vi "LongTimeToShift.vi"(2 "input string":string) -> (0 "s? t:f":string)   [LabVIEW 2012]
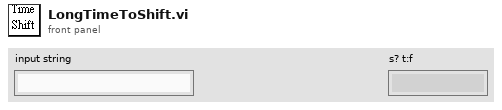
[diagram p1: front panel]
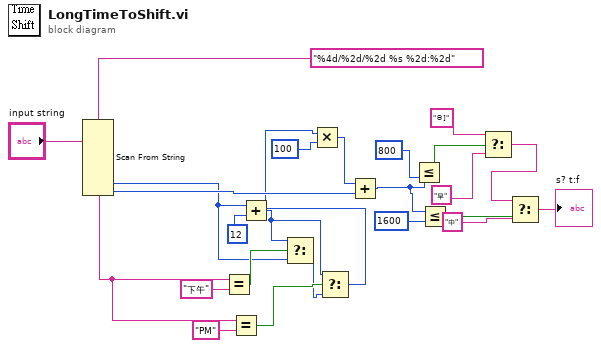
[diagram p0: block diagram]
diagram:
  n1 = Scan From String(format string="%4d/%2d/%2d %s %2d:%2d", input string="input string") -> (output 4=w5:string, output 5=w7:i32, output 6=w11:i32)  [unwired: 11 in, 3 out]
  n2 = Equal?(x=w5, y="下午") -> (x = y?=w9:bool)
  n3 = Equal?(x=w5, y="PM") -> (x = y?=w4:bool)
  n4 = Add(x=w7, y=12) -> (x+y=w2:i32)
  n5 = Select(t=w2, s=w9, f=w7) -> (s? t:f=w1:i32)
  n6 = Select(t=w2, s=w4, f=w1) -> (s? t:f=w3:i32)
  n7 = Multiply(x=w3, y=100) -> (x*y=w23:i32)
  n8 = Add(x=w23, y=w11) -> (x+y=w13:i32)
  n9 = Less Or Equal?(x=w13, y=800) -> (x <= y?=w21:bool)
  n10 = Less Or Equal?(x=w13, y=1600) -> (x <= y?=w17:bool)
  n11 = Select(t="©]", s=w21, f="早") -> (s? t:f=w12:string)
  n12 = Select(t=w12, s=w17, f="中") -> (s? t:f=→"s? t:f":string)
